vi "svx_Polar_Draw_Angle_Lines.vi"(6 "probe angle [deg]":u16, 8 "grid measurements":T1 {"end angle" format="%.2f"; "start angle" format="%.2f"; "scale factors"."b" format="%.2f"; "scale factors"."a" format="%.2f"}, 9 "decade specs":cluster{"radius":i16, "label":string}[](array[cluster]), 11 "picture":picture) -> (3 "new picture":picture)   [LabVIEW 2017, in "SVX Polar Plot.xctl"]
uses:
  <vilib>/addons/_XControls/Polar Plot/SVX Polar Plot.xctl
panel:
  in  "?":cluster{"angle":dbl, "min radius":i16}[](array[cluster])=[{"angle"=0.0, "min radius"=0}, {"angle"=15.0, "min radius"=25}, {"angle"=30.0, "min radius"=25}, {"angle"=45.0, "min radius"=10}, {"angle"=60.0, "min radius"=25}, {"angle"=75.0, "min radius"=25}] {"angle" format="%.2f"}
  # "To change the number of\nangle lines drawn add or\nremove elements from\nthis array.  (Changes\nwill only be temporary\nunless you make the new\nvalue the default and save\nthe VI.)\n\nAngle refers to the angle\nof the line in degrees.  The\nangles should be >=0 and\n<90, as these values are\nrepeated for each quadrant.\n\nMin radius refers to the\nsmallest size circle the\nlines should be drawn to."
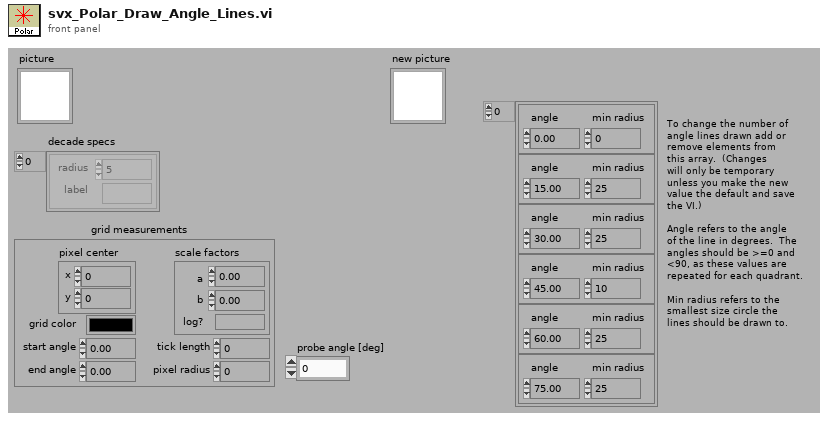
[diagram p1: front panel]
types:
  T1 = cluster{"pixel center":cluster{"x":i16, "y":i16}, "scale factors":cluster{"a":dbl, "b":dbl, "log?":bool}, "grid color":u32, "start angle":dbl, "end angle":dbl, "tick length":i16, "pixel radius":i32}
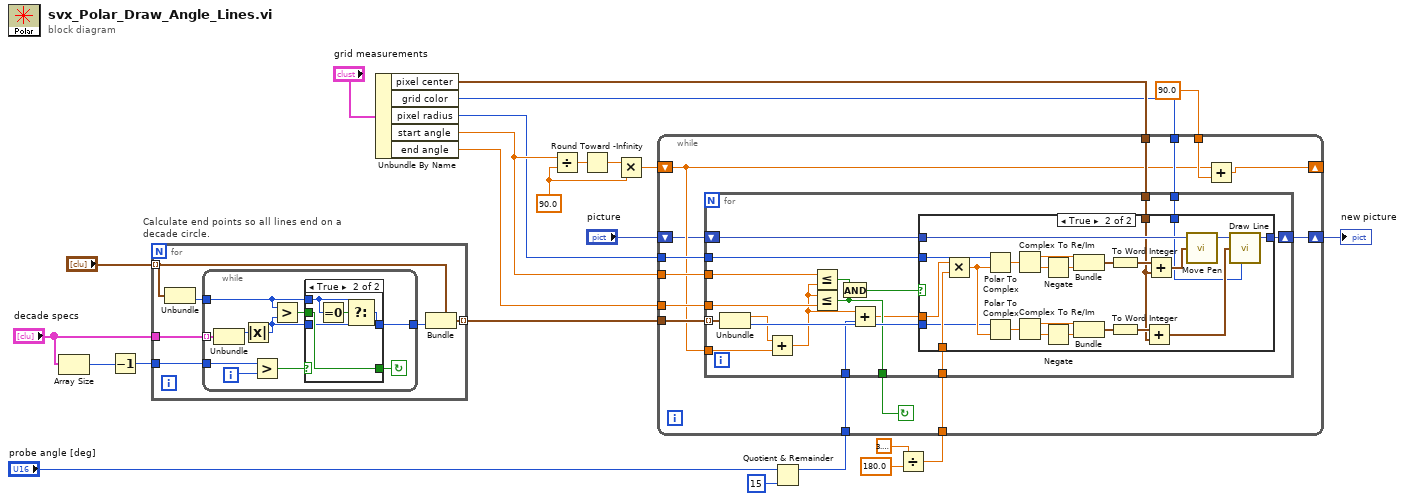
[diagram p0: block diagram]
diagram:
  w6 = 90.0
  n1 = Array Size(array="decade specs") -> (size(s)=w1:i32)
  n2 = Decrement(x=w1) -> (x-1=w2:i32)
  n3 = for "Calculate end points so all lines end on a decade circle." {
    tunnel: "?" -> [w27] mode=indexing
    tunnel: "decade specs" -> [w30]
    tunnel: w2 -> [w29]
    tunnel: [w25] -> w11 mode=indexing
    n4 = Unbundle(w27) -> ("min radius"=w28:i16)  [unwired: 1 out]
    n5 = while {
      tunnel: [w33] -> w26
      tunnel: w28 -> [w32]
      tunnel: w29 -> [w38]
      tunnel: w30 -> [w40] mode=indexing
      i -> [w39]
      stop <- w36 continue-if-true
      n6 = Unbundle(w40) -> ("radius"=w35:i16)  [unwired: 1 out]
      n7 = Absolute Value(x=w35) -> (abs(x)=w31:i16)
      n8 = Greater?(x=w38, y=w39) -> (0:w37:bool)
      n9 = Greater?(x=w32, y=w31) -> (0:w34:bool)
      n10 = case shown="True" w37 {
        selector: w37 -> [w42 _]
        tunnel: [w42 w47] -> w36
        tunnel: w31 -> [w41 w43]
        tunnel: w34 -> [_ w47]
        tunnel: [w41 w44] -> w33
        tunnel: w32 -> [_ w45]
        frame False {
          # "last element"
        }
        frame True {
          n11 = Equal To 0?(x=w45) -> (x = 0?=w46:bool)
          n12 = Select(t=w45, s=w46, f=w43) -> (s? t:f=w44:i16)
        }
      }
    }
    n13 = Bundle(cluster=w27, "min radius"=w26) -> (w25:cluster{"angle":dbl, "min radius":i16})  [unwired: 1 in]
  }
  n14 = Unbundle By Name("grid measurements") -> ("pixel center"=w23:cluster{"x":i16, "y":i16}, "grid color"=w10:u32, "pixel radius"=w12:i32, "start angle"=w14:dbl, "end angle"=w13:dbl)
  n15 = Divide(x=w14, y=w6) -> (x/y=w18:dbl)
  n16 = Round Toward -Infinity(1:w18) -> (0:w17:dbl)
  n17 = Multiply(x=w17, y=w6) -> (x*y=w16:dbl)
  n18 = Quotient & Remainder(x="probe angle [deg]", y=u16 15) -> (x-y*floor(x/y)=w4:u16)  [unwired: 1 out]
  n19 = Divide(x=3.141592653589793, y=180.0) -> (x/y=w15:dbl)
  n20 = while {
    shift-left: "picture" -> [w50]
    shift-right: [w49] -> w8
    tunnel: 90.0 -> [w53]
    tunnel: w10 -> [w54]
    tunnel: w23 -> [w55]
    tunnel: w11 -> [w56]
    tunnel: w12 -> [w57]
    tunnel: w13 -> [w58]
    tunnel: w14 -> [w59]
    tunnel: w15 -> [w60]
    shift-left: w16 -> [w52]
    shift-right: [w61] -> _
    tunnel: w4 -> [w48]
    stop <- w51 continue-if-true
    n21 = for {
      tunnel: w56 -> [w79] mode=indexing
      shift-right: [w77] -> w49
      shift-left: w50 -> [w78]
      tunnel: w55 -> [w76]
      tunnel: w54 -> [w75]
      tunnel: w60 -> [w74]
      tunnel: w59 -> [w70]
      tunnel: w58 -> [w69]
      tunnel: w57 -> [w68]
      tunnel: w52 -> [w67]
      tunnel: [w65] -> w51
      tunnel: w48 -> [w64]
      n22 = Unbundle(w79) -> ("angle"=w66:dbl, "min radius"=w73:i16)
      n23 = Add(x=w66, y=w67) -> (x+y=w63:dbl)
      n24 = Less Or Equal?(x=w70, y=w63) -> (x <= y?=w72:bool)
      n25 = Less Or Equal?(x=w63, y=w69) -> (x <= y?=w65:bool)
      n26 = And(x=w72, y=w65) -> (x .and. y?=w71:bool)
      n27 = Add(x=w63, y=w64) -> (x+y=w62:dbl)
      n28 = case shown="True" w71 {
        tunnel: w78 -> [w80 w90]
        tunnel: [w80 w89] -> w77
        tunnel: w76 -> [_ w88]
        tunnel: w75 -> [_ w87]
        tunnel: w68 -> [_ w86]
        tunnel: w74 -> [_ w85]
        tunnel: w73 -> [_ w84]
        tunnel: w62 -> [_ w83]
        frame False {
        }
        frame True {
          n29 = Multiply(x=w83, y=w85) -> (x*y=w97:dbl)
          n30 = Polar To Complex(1:w97, 2:w86) -> (0:w96:cdb)
          n31 = Polar To Complex(1:w97, 2:w84) -> (0:w93:cdb)
          n32 = Complex To Re/Im(x + iy=w96) -> (x=w98:dbl, y=w99:dbl)
          n33 = Complex To Re/Im(x + iy=w93) -> (x=w94:dbl, y=w95:dbl)
          n34 = Negate(x=w99) -> (-x=w81:dbl)
          n35 = Negate(x=w95) -> (-x=w82:dbl)
          n36 = Bundle(w98, w81) -> (w91:cluster{dbl, dbl})  [unwired: 1 in]
          n37 = Bundle(w94, w82) -> (w92:cluster{dbl, dbl})  [unwired: 1 in]
          n38 = To Word Integer(number=w91) -> (16bit integer=w101:cluster{i16, i16})
          n39 = To Word Integer(number=w92) -> (16bit integer=w100:cluster{i16, i16})
          n40 = Add(x=w100, y=w88) -> (x+y=w104:cluster{i16, i16})
          n41 = Add(x=w101, y=w88) -> (x+y=w103:cluster{i16, i16})
          n42 = call <vilib>:"Move Pen.vi"("new position"=w103, "picture"=w90) -> ("new picture"=w102:picture)  [unwired: 3 in]
          n43 = call <vilib>:"Draw Line.vi"("picture"=w102, "end point"=w104, "color(black)"=w87) -> ("new picture"=w89:picture)  [unwired: 6 in]
        }
      }
    }
    n44 = Add(x=w52, y=w53) -> (x+y=w61:dbl)
  }
  "new picture" <- w8
